vi "Test Opened Config Stays Open on Boolean Read.vi"(8 "error in (no error)":errorcluster, 11 "Test Case In":refnum<class "Configuration File Reference Management Test.lvclass">) -> (0 "error out":errorcluster, 3 "Test Case Out":refnum<class "Configuration File Reference Management Test.lvclass">)   [LabVIEW 2020, in "Configuration File Reference Management Test.lvclass"]
uses:
  Configuration File Reference Management Test.lvclass
  C:/Program Files (x86)/National Instruments/LabVIEW 2020/vi.lib/Astemes/LUnit/Test Case.lvclass
  Mock Configurable Base/Mock Configurable Base.lvclass
  <vilib>/Astemes/LUnit/Test Case.lvclass/Test Case.ctl
  <vilib>/Astemes/LUnit/Palette/Fail.vi
  <vilib>/Astemes/LUnit/Palette/Pass.vi
  <vilib>/Astemes/LUnit/Set Assertion Type.vi
  <vilib>/Astemes/LUnit/Add test result.vi
  <vilib>/Astemes/LUnit/LUnit Record Assertion Result.vi
  <vilib>/Astemes/LUnit/LUnit Aggregate Assertion Results.vi
  <vilib>/Astemes/LUnit/Method Result/LUnit Merge Status.vi
  <vilib>/Astemes/LUnit/LUnit Concatenate result strings.vi
  Configuration File Reference Management Test.lvclass/Configuration File Reference Management Test.ctl
  <vilib>/Astemes/LUnit/Test Case.lvclass
  C:/Git/astemes-triarc-framework/tests/Configuration File Reference Management Test/Configuration File Reference Management Test.lvclass
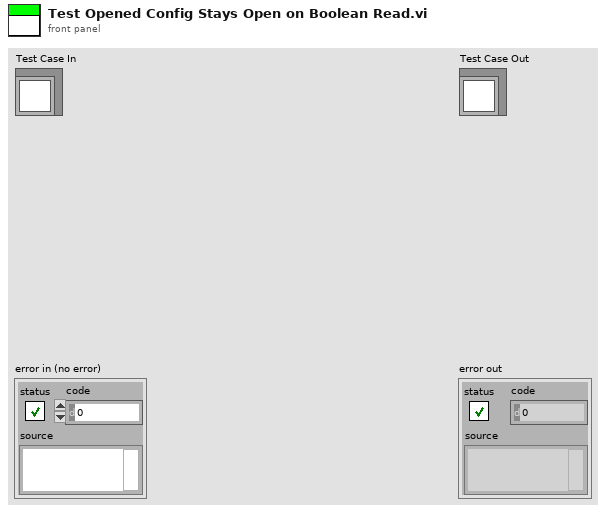
[diagram p1: front panel]
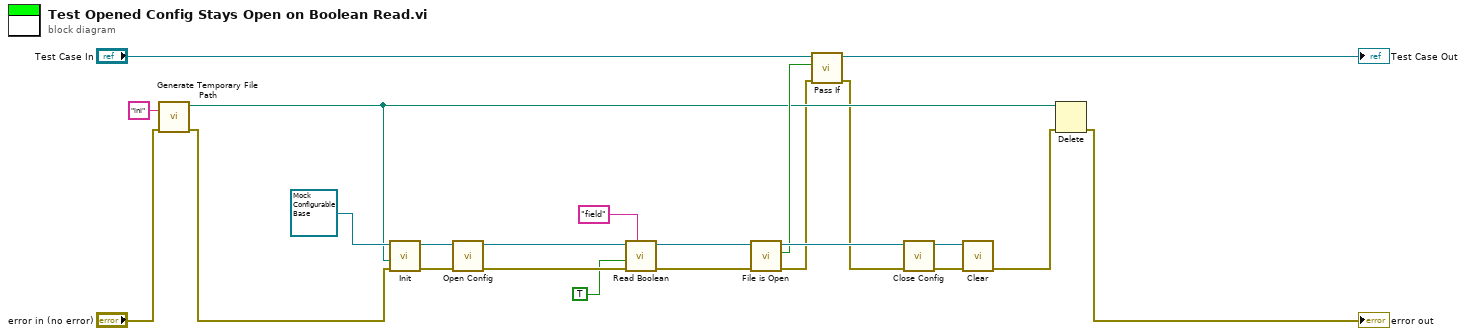
[diagram p0: block diagram]
diagram:
  n1 = call <vilib>:"Generate Temporary File Path.vi"("error in (no error)"="error in (no error)", "Temporary File Extension (tmp)"="ini") -> ("error out"=w21:errorcluster, "Unique Temporary File Path"=w5:path)  [unwired: 8 in]
  n2 = call-dynamic "Init.vi"("error in (no error)"=w21, "Config File Path"=w5, "Base In"=refnum<class "Mock Configurable Base.lvclass"> refnum ("Mock Configurable Base.lvclass")) -> ("error out"=w15:errorcluster, "Base Out"=w16:refnum<class "Mock Configurable Base.lvclass">)  [unwired: 7 in]
  n3 = call-dynamic "Open Config.vi"("error in (no error)"=w15, "Configuration File File In"=w16) -> ("error out"=w19:errorcluster, "Configuration File File Out"=w18:refnum<class "Mock Configurable Base.lvclass">)  [unwired: 8 in]
  n4 = call-dynamic "Read Boolean.vi"("key"="field", "error in (no error)"=w19, "default value"=TRUE ("Value"), "Configuration File In"=w18) -> ("error out"=w14:errorcluster, "Configuration File Out"=w9:refnum<class "Mock Configurable Base.lvclass">)  [unwired: 5 in, 1 out]
  n5 = call "File is Open.vi"("error in (no error)"=w14, "Mock Configurable Base in"=w9) -> ("error out"=w2:errorcluster, "Is open?"=w6:bool, "Mock Configurable Base out"=w8:refnum<class "Mock Configurable Base.lvclass">)  [unwired: 7 in]
  n6 = call <vilib>:"Pass If.vi"("error in (no error)"=w2, "Pass?"=w6, "LUnit Test Case In"="Test Case In") -> ("error out"=w1:errorcluster, "LUnit Test Case Out"=→"Test Case Out":refnum<class "Configuration File Reference Management Test.lvclass">)  [unwired: 7 in]
  n7 = call-dynamic "Close Config.vi"("error in (no error)"=w1, "Configuration File File In"=w8) -> ("error out"=w12:errorcluster, "Configuration File File Out"=w13:refnum<class "Mock Configurable Base.lvclass">)  [unwired: 8 in]
  n8 = call-dynamic "Clear.vi"("error in (no error)"=w12, "Base In"=w13) -> ("error out"=w4:errorcluster)  [unwired: 9 in]
  n9 = Delete(path (use dialog)=w5, error in=w4) -> (error out=→"error out":errorcluster)  [unwired: 3 in, 2 out]
